vi "Send frame rate.vi"(8 "error in (no error)":errorcluster, 11 "DAQOrcaFlash in":refnum<class "DAQOrcaFlash.lvclass">) -> (0 "error out":errorcluster, 3 "DAQOrcaFlash out":refnum<class "DAQOrcaFlash.lvclass">)   [LabVIEW 2012, in "DAQOrcaFlash.lvclass"]
uses:
  DAQOrcaFlash.lvclass
  <vilib>/Distrio/Murmex/Murmex/Murmex.lvclass
  <vilib>/Distrio/Murmex/Murmex/update_cluster.ctl
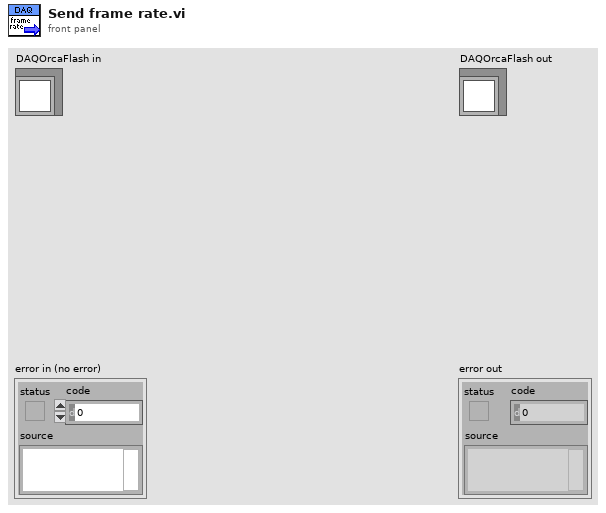
[diagram p1: front panel]
types:
  T1 = typedef "Murmex.lvlib/Murmex.lvclass/update_cluster.ctl" = cluster{"target ID":string, "key chains":string[], "values":variant[]}
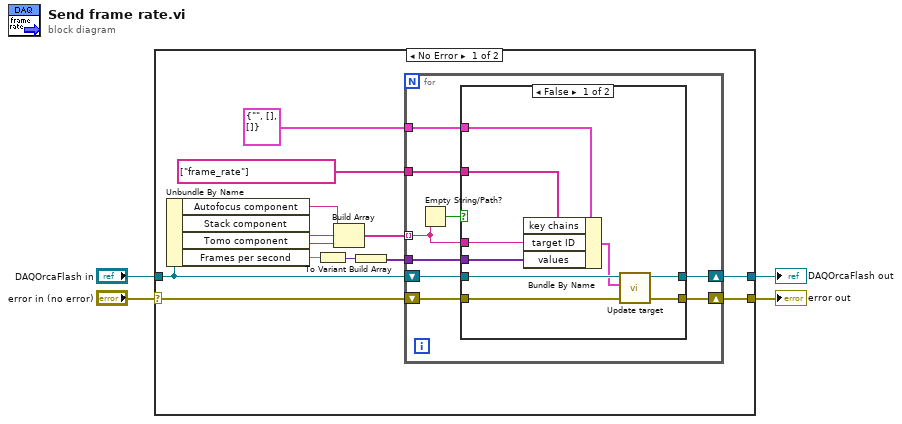
[diagram p0: block diagram]
diagram:
  n1 = case shown="No Error" "error in (no error)" {
    selector: "error in (no error)" -> [w17 w38]
    tunnel: [w16 w38] -> w1
    tunnel: [w14 w39] -> w2
    tunnel: "DAQOrcaFlash in" -> [w15 w39]
    frame No Error {
      n2 = Unbundle By Name(w15) -> ("Autofocus component"=w5:string, "Stack component"=w9:string, "Tomo component"=w10:string, "Frames per second"=w13:dbl[unit])
      n3 = To Variant(anything=w13) -> (Variant=w12:variant)
      n4 = Build Array(w5, w9, w10) -> (w8:string[])
      n5 = Build Array(w12) -> (w11:variant[])
      n6 = for {
        tunnel: w11 -> [w22]
        tunnel: w8 -> [w19] mode=indexing
        tunnel: string[] ["frame_rate"] ("key chains") -> [w21]
        tunnel: T1 {"target ID"="", "key chains"=[], "values"=[]} ("update cluster") -> [w20]
        shift-right: [w25] -> w16
        shift-left: w17 -> [w26]
        shift-right: [w23] -> w14
        shift-left: w15 -> [w24]
        n7 = Empty String/Path?(string/path=w19) -> (empty?=w18:bool)
        n8 = case shown="False" w18 {
          tunnel: w26 -> [w35 w36]
          tunnel: [w34 w36] -> w25
          tunnel: w24 -> [w33 w37]
          tunnel: [w32 w37] -> w23
          tunnel: w22 -> [w31 _]
          tunnel: w21 -> [w30 _]
          tunnel: w20 -> [w29 _]
          tunnel: w19 -> [w27 _]
          frame False {
            n9 = Bundle By Name(cluster=w29, "key chains"=w30, "target ID"=w27, "values"=w31) -> (w28:T1)
            n10 = call <vilib>:"Update target.vi"("error in (no error)"=w35, "update cluster"=w28, "MurmexBase in"=w33) -> ("error out"=w34:errorcluster, "MurmexBase out"=w32:refnum<class "DAQOrcaFlash.lvclass">)  [unwired: 7 in]
          }
          frame True {
          }
        }
      }
    }
    frame Error {
    }
  }
  "error out" <- w1
  "DAQOrcaFlash out" <- w2
